vi "Map Global Variables.vi"() -> ()   [LabVIEW 2011]
panel:
  in  "End Program":bool
  in  "Map Data":T1={"X"=350.0, "Y"=570.0, "Zoom"=15.0, "Map Format"="roadmap", "Google Maps API Key"="AIzaSyDQES5BW68QG5HzTQIG5gxZIUTr_OVHJhg", "Map Refresh Rate (milliseconds)"=5000} {"Zoom" format="%#.1g"}
  in  "Boundary Data":T2={"Path Color"=16715776, "Weight"=5, "Path Data"=[]} {"Path Data"."Final Latitude" format="%#.6g"; "Path Data"."Final Longitude" format="%#.6g"; "Path Data"."Initial Longitude" format="%#.6g"; "Path Data"."Initial Latitude" format="%#.6g"}
  in  "Navigation Data":T3={"Balloon Color"="purple", "Balloon Size"="mid", "Navigation Waypoints"=[]} {"Navigation Waypoints"."Longitude" format="%#.6g"; "Navigation Waypoints"."Latitude" format="%#.6g"}
  in  "Current Location Data":cluster{"Lat":dbl, "Lon":dbl}={"Lat"=51.4062, "Lon"=-1.3070000000000026} {"Lon" format="%#.6g"; "Lat" format="%#.6g"}
  out "URL":string="http://maps.google.com/staticmap?center=51.406200,-1.307000&zoom=18&size=570x350&maptype=hybrid&markers=51.406200,-1.307000,midpurplea&key=&path=rgb:0xFF1000,weight:5|51.406200,-1.307000|51.406200,-1.307000"
  in  "Map":refnum<k7>(container)
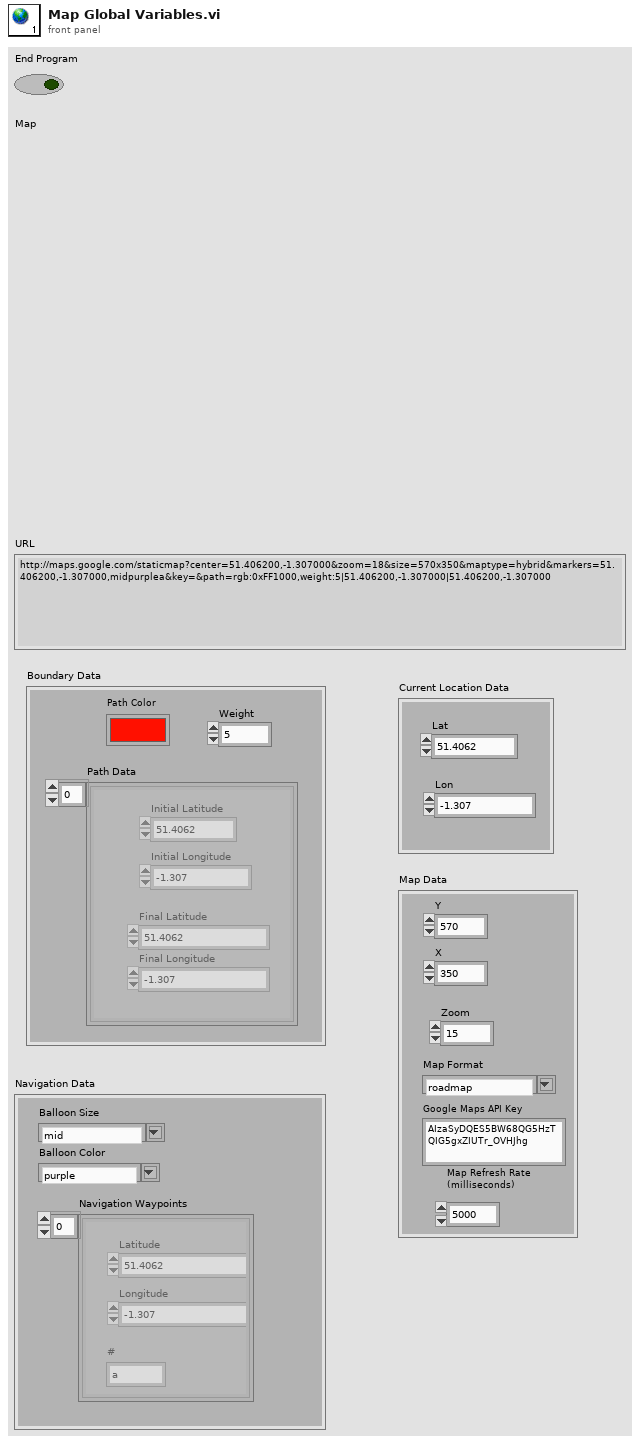
[diagram p1: front panel]
types:
  T1 = cluster{"X":dbl, "Y":dbl, "Zoom":sgl, "Map Format":string, "Google Maps API Key":string, "Map Refresh Rate (milliseconds)":u32}
  T2 = cluster{"Path Color":u32, "Weight":i32, "Path Data":cluster{"Initial Latitude":dbl, "Initial Longitude":dbl, "Final Longitude":dbl, "Final Latitude":dbl}[]}
  T3 = cluster{"Balloon Color":string, "Balloon Size":string, "Navigation Waypoints":cluster{"#":string, "Latitude":dbl, "Longitude":dbl}[]}
diagram:
